vi "Begin.vi"(8 "error in":errorcluster) -> (0 "error out":errorcluster)   [LabVIEW 2020]
doc: "Called before other user functions, this VI is expected to open initial I/O refnums, load in file data, and do all program initialization. Notice that the <B>error out</B> terminal is simply used for data flow. Wiring it to other structures or subVIs ensures that this VI runs first."
uses:
  <vilib>/Rock Robotics/WPI/ThirdParty/Phoenix-LabVIEW/Pigeon2/controls/CTRE_Phoenix_Pigeon2_Configurables.ctl
  <vilib>/Rock Robotics/WPI/DriverStation/WPI_DriverStationRobotMode2.ctl
  <vilib>/Rock Robotics/WPI/Joystick/WPI_JoystickDeviceEnum.ctl
  <vilib>/Rock Robotics/WPI/SafetyOutput/WPI_SafetyOutputConfigMenu.ctl
  <vilib>/Rock Robotics/SystemInterfaces/DIO/FPGA_DIOChannel.ctl
  <vilib>/Rock Robotics/WPI/Solenoid/WPI_SolenoidChannel.ctl
  Robot Global Data.vi
  <vilib>/Rock Robotics/Network Tables/NT Write String Array.vi
  <vilib>/Rock Robotics/WPI/RobotDrive/WPI_RobotDriveOpen2MotorWithExistingMotors.vi
  <vilib>/Rock Robotics/WPI/Switch/WPI_SwitchOpenLimit.vi
  <vilib>/Rock Robotics/WPI/Solenoid/WPI_SolenoidOpenDouble.vi
panel:
  in  "Pigeon2 Configurables":T1
  in  "error in 2":errorcluster
  out "error out 2":errorcluster
  # "Yaw Angle needed to reach the current orientation in degrees"
  # "Configures the mounting pose of the Pigeon2\nThis is the yaw-pitch-roll teh Pigeon2 underwent to get to its current orientation,\n referenced from the robot's point of view\nThis is only necessary if the Pigeon2 is mounted at an exotic angle near the gimbal lock point or not forward.\nIf the pigeon is relatively flat and pointed forward, this is not needed"
  # "Pitch Angle needed to reach the current orientation in degrees"
  # "Roll Angle needed to reach the current orientation in degrees"
  # "Disables the temperature compensation\nfrom the Pigeon2. It is recommended that\nthis remains false"
  # "Disables the no-motion calibration from the\nPigeon2. It is recommended that this \nremains false"
  # "Enables the compass for Pigeon2\nThis is not recommended for any indoor robotics"
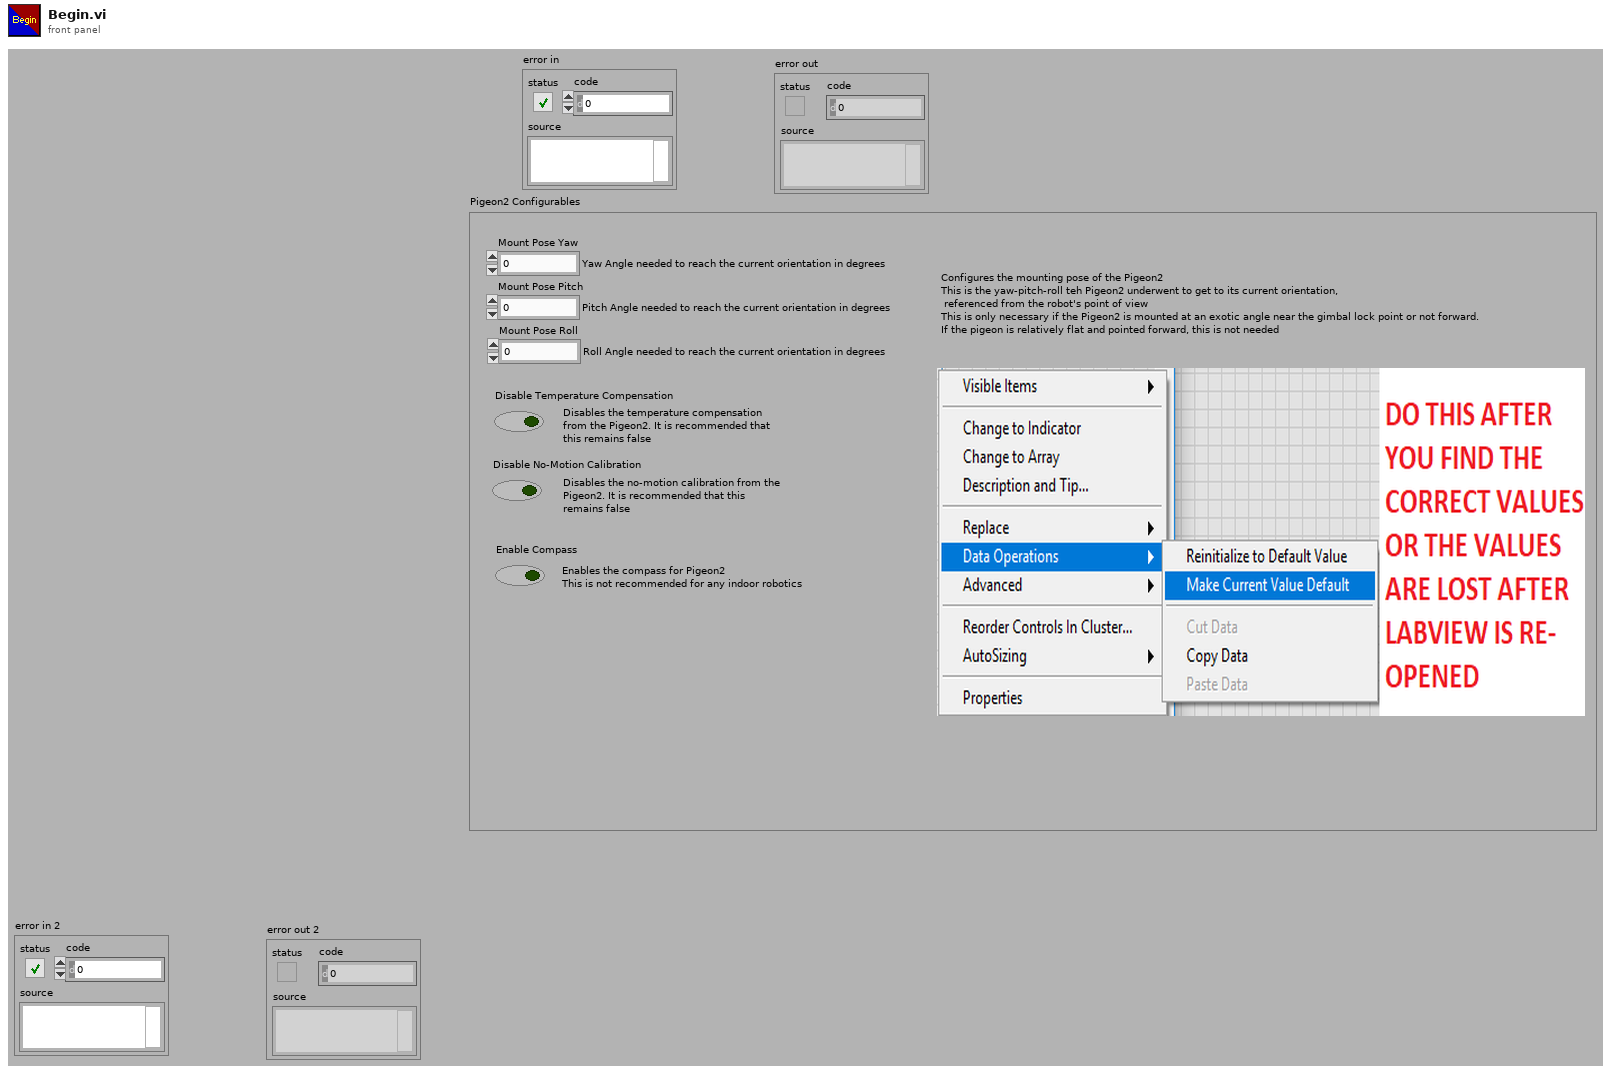
[diagram p1: front panel]
types:
  T1 = typedef "CTRE_Phoenix_Pigeon2_Configurables.ctl" = cluster{"Mount Pose Yaw":dbl, "Mount Pose Pitch":dbl, "Mount Pose Roll":dbl, "Disable Temperature Compensation":bool, "Disable No-Motion Calibration":bool, "Enable Compass":bool}
  T2 = typedef "WPI_SolenoidChannel.ctl" = enum8{"Solenoid 0", "Solenoid 1", "Solenoid 2", "Solenoid 3", "Solenoid 4", "Solenoid 5", "Solenoid 6", "Solenoid 7", "Solenoid 8", "Solenoid 9", "Solenoid 10", "Solenoid 11", "Solenoid 12", "Solenoid 13", "Solenoid 14", "Solenoid 15", "Invalid"}
  T3 = typedef "FPGA_DIOChannel.ctl" = enum8{"DIO 0", "DIO 1", "DIO 2", "DIO 3", "DIO 4", "DIO 5", "DIO 6", "DIO 7", "DIO 8", "DIO 9", "DIO MXP 0", "DIO MXP 1", "DIO MXP 2", "DIO MXP 3", "DIO MXP 4", "DIO MXP 5", "DIO MXP 6", "DIO MXP 7", "DIO MXP 8", "DIO MXP 9", "DIO MXP 10", "DIO MXP 11", "DIO MXP 12", "DIO MXP 13", "DIO MXP 14", "DIO MXP 15", "SPI Port CS1", "SPI Port CS2", "SPI Port CS3", "SPI Port MISO", "SPI Port MOSI", "Invalid"}
  T4 = typedef "WPI_JoystickDeviceEnum.ctl" = enum16{"USB 0", "USB 1", "USB 2", "USB 3", "USB 4", "USB 5"}
  T5 = typedef "WPI_SafetyOutputConfigMenu.ctl" = enum16{"Enable", "Disable"}
  T6 = typedef "WPI_DriverStationRobotMode2.ctl" = enum16{"Autonomous Disabled", "Autonomous Enabled", "Teleop Disabled", "Teleop Enabled", "Disconnected", "Finish", "Test Disabled", "Test Enabled", "Emergency Stopped"}
  T7 = typedef "WPI_JoystickDevRef.ctl" = cluster{"Device":T4}
  T8 = typedef "CTRE_PigeonIMU_DeviceRef.ctl" = cluster{"DeviceStatus":errorcluster, "Device Number":u8, "Type":T9, "Device ID":u32, "Handle":u64, "UsageFrame":u32, "Library Path":path}
  T9 = typedef "CTRE_PigeonIMU_ConnectionType.ctl" = u32
  T10 = typedef "WPI_SwitchDevRef.ctl" = cluster{"DevStatus":errorcluster, "DIO Channel":T3, "CntIndex":T11, "Normally Closed":bool}
  T11 = typedef "FPGA_CounterCtrSystemIndex.ctl" = enum8{"Ctr 0", "Ctr 1", "Ctr 2", "Ctr 3", "Ctr 4", "Ctr 5", "Ctr 6", "Ctr 7", "Invalid"}
  T12 = typedef "WPI_MotorControlDeviceRef.ctl" = cluster{"DeviceStatus":errorcluster, "Type":T13, "PWM":cluster{"PWM Channel":T14, "DeadBand":T15}, "CAN":cluster{"Device Number":u8, "SetOutput VI Ref":variant, "GetOutput VI Ref":variant, "Enable VI Ref":variant, "Disable VI Ref":variant, "Data":variant}, "Invert":bool, "DIO PWM":cluster{"PWM \"Enable\" Channel":T14, "DIOChannel":T3, "PWM Rate":dbl}}
  T13 = typedef "WPI_MotorControlType.ctl" = enum16{"PWM", "CAN", "DIO PWM"}
  T14 = typedef "FPGA_DIOPWMChannel.ctl" = enum8{"PWM 0", "PWM 1", "PWM 2", "PWM 3", "PWM 4", "PWM 5", "PWM 6", "PWM 7", "PWM 8", "PWM 9", "PWM MXP 0", "PWM MXP 1", "PWM MXP 2", "PWM MXP 3", "PWM MXP 4", "PWM MXP 5", "PWM MXP 6", "PWM MXP 7", "PWM MXP 8", "PWM MXP 9", "Invalid"}
  T15 = typedef "WPI_PWMDeadband.ctl" = cluster{"Name":string, "maxPositivePwm":i32, "minPositivePwm":i32, "centerPwm":i32, "maxNegativePwm":i32, "minNegativePwm":i32, "angularRange":u16}
  T16 = typedef "WPI_RobotDriveDevRef.ctl" = cluster{"DevStatus":errorcluster, "Motors[]":T12[], "Square Inputs":bool, "Max Output":dbl}
  T17 = typedef "WPI_SolenoidDevRef.ctl" = cluster{"DevStatus":errorcluster, "Pneumatics Control Module":u8, "Forward Solenoid Channel":T2, "Reverse Solenoid Channel":T2}
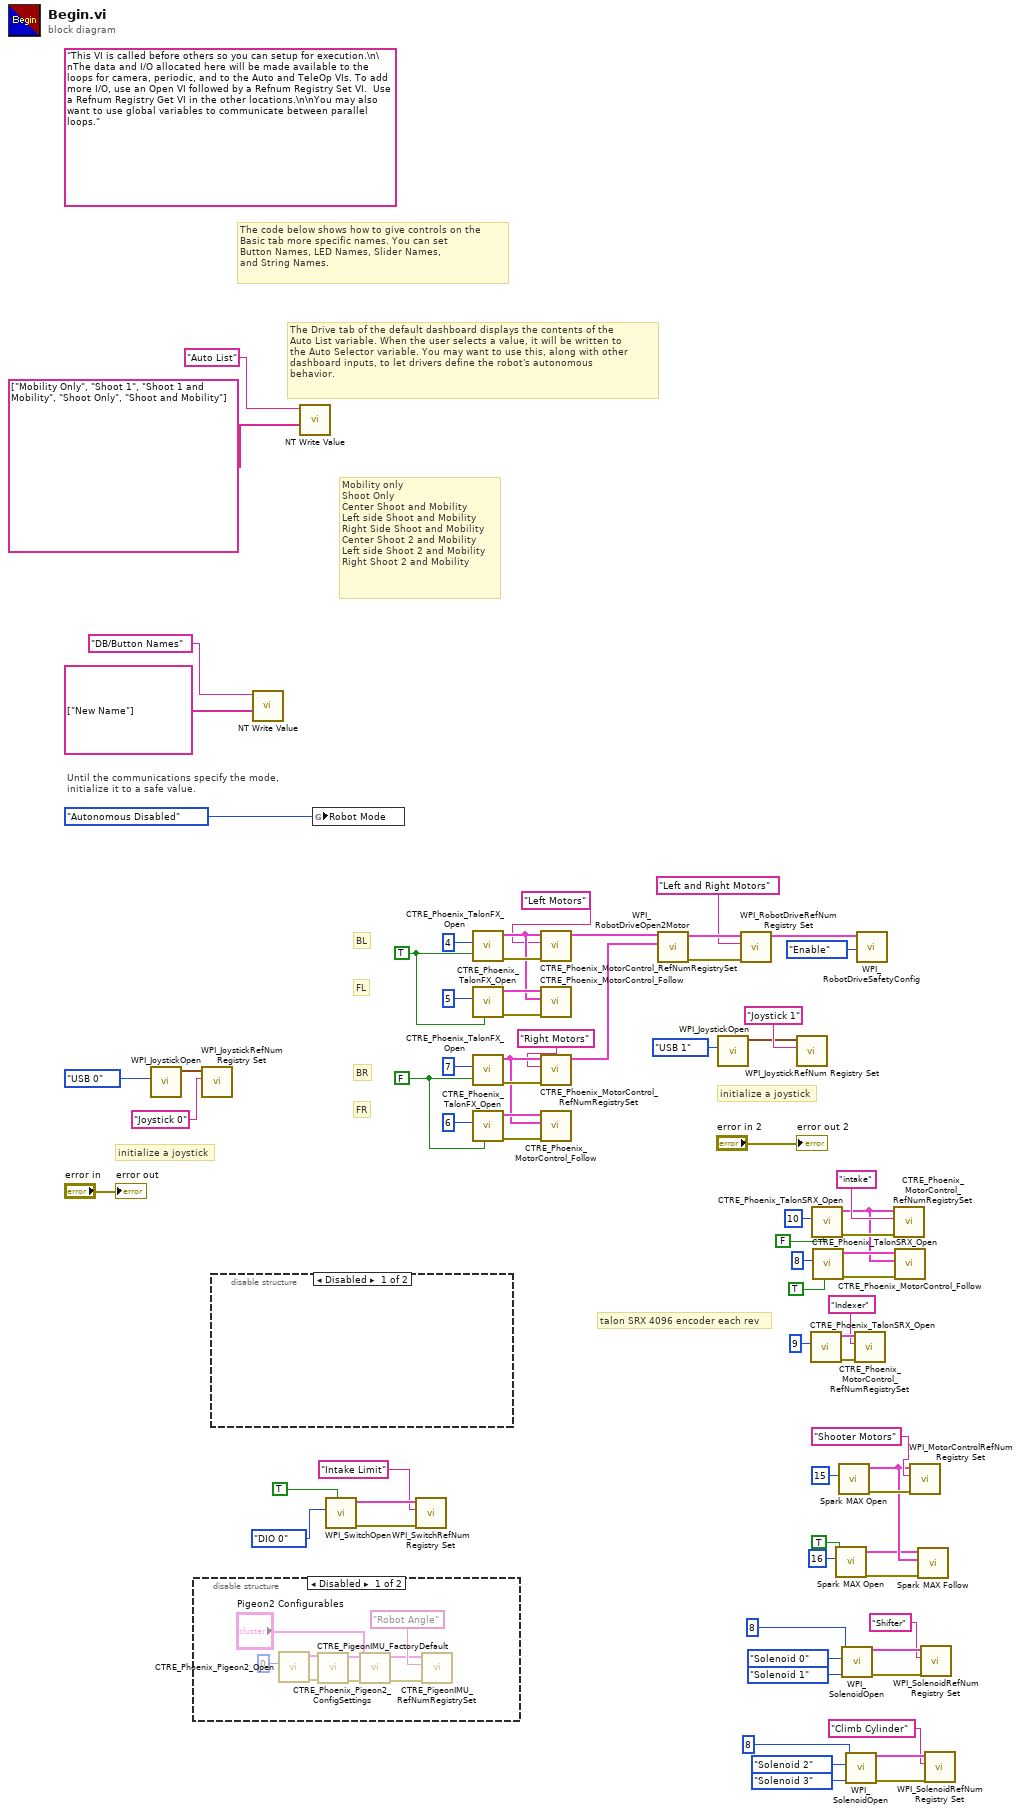
[diagram p0: block diagram]
diagram:
  w21 = TRUE ("Invert")
  w22 = FALSE ("Invert")
  (unwired) "This VI is called before others so you can setup for execution.\n\nThe data and I/O allocated here will be made available to the loops for camera, periodic, and to the Auto and TeleOp VIs. To add more I/O, use an Open VI followed by a Refnum Registry Set VI.  Use a Refnum Registry Get VI in the other locations.\n\nYou may also want to use global variables to communicate between parallel loops."
  # "Mobility only\nShoot Only\nCenter Shoot and Mobility\nLeft side Shoot and Mobility\nRight Side Shoot and Mobility\nCenter Shoot 2 and Mobility\nLeft side Shoot 2 and Mobility\nRight Shoot 2 and Mobility"
  # "talon SRX 4096 encoder each rev"
  # "FL"
  # "BL"
  # "BR"
  # "FR"
  # "initialize a joystick"
  # "The Drive tab of the default dashboard displays the contents of the\nAuto List variable. When the user selects a value, it will be written to\nthe Auto Selector variable. You may want to use this, along with other\ndashboard inputs, to let drivers define the robot's autonomous\nbehavior."
  # "The code below shows how to give controls on the\nBasic tab more specific names. You can set\nButton Names, LED Names, Slider Names,\nand String Names."
  # "initialize a joystick"
  # "Until the communications specify the mode,\ninitialize it to a safe value."
  n1 = call <vilib>:"WPI_JoystickOpen.vi"("JoystickDevice"=WPI_JoystickDeviceEnum."USB 0") -> ("JoystickDevRef"=w72:T7)  [unwired: 10 in]
  n2 = disable-structure shown="Disabled" {
    frame Disabled {
      n3 = call <vilib>:"CTRE_Phoenix_Pigeon2_Open.vi"("Device Number"=u8 0) -> ("error out"=w76:errorcluster, "PigeonIMUDevRef"=w77:T8)  [unwired: 9 in]
      n4 = call <vilib>:"CTRE_PigeonIMU_FactoryDefault.vi"("error in"=w76, "PigeonIMUDevRef"=w77) -> ("error out"=w78:errorcluster, "PigeonIMUDevRef"=w79:T8)  [unwired: 8 in]
      n5 = call <vilib>:"CTRE_Phoenix_Pigeon2_ConfigSettings.vi"("error in (no error)"=w78, "Pigeon2 Configurables"="Pigeon2 Configurables", "PigeonIMUDevRef 2"=w79) -> ("error out"=w81:errorcluster, "PigeonIMUDevRef"=w82:T8)  [unwired: 7 in]
      n6 = call <vilib>:"CTRE_PigeonIMU_RefNumRegistrySet.vi"("error in (no error)"=w81, "refnum name"="Robot Angle", "PigeonIMUDevRef"=w82) -> ()  [unwired: 7 in, 2 out]
    }
    frame Enabled {
    }
  }
  n7 = call <vilib>:"WPI_JoystickRefNum Registry Set.vi"("refnum name"="Joystick 0", "JoystickDevRef"=w72) -> ()  [unwired: 8 in, 2 out]
  n8 = disable-structure shown="Disabled" {
    frame Disabled {
    }
    frame Enabled {
    }
  }
  n9 = call-poly <vilib>:"NT Write Value.vi"("value"=string[] ["New Name"], "name"="DB/Button Names" ("Name")) -> ()  [unwired: 9 in, 1 out]
  n10 = call-poly <vilib>:"NT Write Value.vi"("value"=string[] ["Mobility Only", "Shoot 1", "Shoot 1 and Mobility", "Shoot Only", "Shoot and Mobility"] ("String Array"), "name"="Auto List" ("Name")) -> ()  [unwired: 9 in, 1 out]
  n11 = global write "Robot Global Data.vi" "Robot Mode"(WPI_DriverStationRobotMode2."Autonomous Disabled" ("Robot Mode")) -> ()
  n12 = call-poly <vilib>:"WPI_SwitchOpen.vi"("Normally Closed"=TRUE, "DIO Channel"=FPGA_DIOChannel."DIO 0") -> ("error out"=w16:errorcluster, "SwitchDevRef"=w17:T10)  [unwired: 8 in]
  n13 = call <vilib>:"WPI_SwitchRefNum Registry Set.vi"("error in (no error)"=w16, "refnum name"="Intake Limit", "SwitchDevRef"=w17) -> ()  [unwired: 7 in, 2 out]
  n14 = call <vilib>:"CTRE_Phoenix_TalonFX_Open.vi"("Invert"=w21, "Device Number"=u8 4) -> ("error out"=w36:errorcluster, "PhoenixMotorControlDevRef"=w34:T12)  [unwired: 8 in]
  n15 = call <vilib>:"CTRE_Phoenix_TalonFX_Open.vi"("Invert"=w21, "Device Number"=u8 5) -> ("error out"=w39:errorcluster, "PhoenixMotorControlDevRef"=w35:T12)  [unwired: 8 in]
  n16 = call <vilib>:"CTRE_Phoenix_TalonFX_Open.vi"("Invert"=w22, "Device Number"=u8 7) -> ("error out"=w30:errorcluster, "PhoenixMotorControlDevRef"=w28:T12)  [unwired: 8 in]
  n17 = call <vilib>:"CTRE_Phoenix_TalonFX_Open.vi"("Invert"=w22, "Device Number"=u8 6) -> ("error out"=w33:errorcluster, "PhoenixMotorControlDevRef"=w29:T12)  [unwired: 8 in]
  n18 = call <vilib>:"CTRE_Phoenix_MotorControl_RefNumRegistrySet.vi"("error in (no error)"=w36, "refnum name"="Left Motors", "PhoenixMotorControlDevRef"=w34) -> ("PhoenixMotorControlDevRef"=w27:T12)  [unwired: 7 in, 1 out]
  n19 = call <vilib>:"CTRE_Phoenix_MotorControl_Follow.vi"("error in (no error)"=w39, "Master Controller to Follow"=w34, "PhoenixMotorControlDevRef"=w35) -> ()  [unwired: 7 in, 2 out]
  n20 = call <vilib>:"CTRE_Phoenix_MotorControl_RefNumRegistrySet.vi"("error in (no error)"=w30, "refnum name"="Right Motors", "PhoenixMotorControlDevRef"=w28) -> ("PhoenixMotorControlDevRef"=w26:T12)  [unwired: 7 in, 1 out]
  n21 = call <vilib>:"CTRE_Phoenix_MotorControl_Follow.vi"("error in (no error)"=w33, "Master Controller to Follow"=w28, "PhoenixMotorControlDevRef"=w29) -> ()  [unwired: 7 in, 2 out]
  n22 = call-poly <vilib>:"WPI_RobotDriveOpen2Motor.vi"("Right Motor Dev Ref"=w26, "Left Motor Dev Ref"=w27) -> ("error out"=w46:errorcluster, "RobotDriveDevRef"=w47:T16)  [unwired: 3 in, 5 out]
  n23 = call <vilib>:"WPI_JoystickOpen.vi"("JoystickDevice"=WPI_JoystickDeviceEnum."USB 1") -> ("JoystickDevRef"=w42:T7)  [unwired: 10 in]
  n24 = call <vilib>:"WPI_RobotDriveRefNum Registry Set.vi"("error in (no error)"=w46, "refnum name"="Left and Right Motors", "RobotDriveDevRef"=w47) -> ("RobotDriveDevRef"=w45:T16)  [unwired: 1 in, 7 out]
  n25 = call <vilib>:"WPI_JoystickRefNum Registry Set.vi"("refnum name"="Joystick 1", "JoystickDevRef"=w42) -> ()  [unwired: 8 in, 2 out]
  n26 = call <vilib>:"CTRE_Phoenix_TalonSRX_Open.vi"("Device Number"=u8 9) -> ("error out"=w57:errorcluster, "PhoenixMotorControlDevRef"=w56:T12)  [unwired: 9 in]
  n27 = call <vilib>:"CTRE_Phoenix_TalonSRX_Open.vi"("Invert"=FALSE, "Device Number"=u8 10) -> ("error out"=w53:errorcluster, "PhoenixMotorControlDevRef"=w20:T12)  [unwired: 8 in]
  n28 = call <vilib>:"CTRE_Phoenix_TalonSRX_Open.vi"("Invert"=TRUE, "Device Number"=u8 8) -> ("error out"=w50:errorcluster, "PhoenixMotorControlDevRef"=w49:T12)  [unwired: 8 in]
  n29 = call <vilib>:"Spark MAX Open.vi"("Invert"=TRUE, "Device Number"=u8 16) -> ("error out"=w59:errorcluster, "MotorControlDeviceRef"=w60:T12)  [unwired: 8 in]
  n30 = call <vilib>:"Spark MAX Open.vi"("Device Number"=u8 15) -> ("error out"=w65:errorcluster, "MotorControlDeviceRef"=w61:T12)  [unwired: 9 in]
  n31 = call-poly <vilib>:"WPI_SolenoidOpen.vi"("Reverse Solenoid Channel"=WPI_SolenoidChannel."Solenoid 1", "Forward Solenoid Channel"=WPI_SolenoidChannel."Solenoid 0", "Pneumatics Device (def)"=u8 8) -> ("error out"=w9:errorcluster, "SolenoidDevRef"=w10:T17)  [unwired: 7 in]
  n32 = call-poly <vilib>:"WPI_SolenoidOpen.vi"("Reverse Solenoid Channel"=WPI_SolenoidChannel."Solenoid 3", "Forward Solenoid Channel"=WPI_SolenoidChannel."Solenoid 2", "Pneumatics Device (def)"=u8 8) -> ("error out"=w4:errorcluster, "SolenoidDevRef"=w5:T17)  [unwired: 7 in]
  n33 = call <vilib>:"CTRE_Phoenix_MotorControl_RefNumRegistrySet.vi"("error in (no error)"=w57, "refnum name"="Indexer", "PhoenixMotorControlDevRef"=w56) -> ()  [unwired: 7 in, 2 out]
  n34 = call <vilib>:"WPI_RobotDriveSafetyConfig.vi"("mode"=WPI_SafetyOutputConfigMenu."Enable", "RobotDriveDevRef"=w45) -> ()  [unwired: 8 in, 2 out]
  n35 = call <vilib>:"CTRE_Phoenix_MotorControl_RefNumRegistrySet.vi"("error in (no error)"=w53, "refnum name"="intake", "PhoenixMotorControlDevRef"=w20) -> ()  [unwired: 7 in, 2 out]
  n36 = call <vilib>:"CTRE_Phoenix_MotorControl_Follow.vi"("error in (no error)"=w50, "Master Controller to Follow"=w20, "PhoenixMotorControlDevRef"=w49) -> ()  [unwired: 7 in, 2 out]
  n37 = call <vilib>:"WPI_MotorControlRefNum Registry Set.vi"("error in (no error)"=w65, "refnum name"="Shooter Motors", "MotorControlDevRef"=w61) -> ()  [unwired: 7 in, 2 out]
  n38 = call <vilib>:"Spark MAX Follow.vi"("error in (no error)"=w59, "Master Controller"=w61, "MotorControlDeviceRef"=w60) -> ()  [unwired: 7 in, 2 out]
  n39 = call <vilib>:"WPI_SolenoidRefNum Registry Set.vi"("error in (no error)"=w9, "refnum name"="Shifter", "SolenoidDevRef"=w10) -> ()  [unwired: 7 in, 2 out]
  n40 = call <vilib>:"WPI_SolenoidRefNum Registry Set.vi"("error in (no error)"=w4, "refnum name"="Climb Cylinder", "SolenoidDevRef"=w5) -> ()  [unwired: 7 in, 2 out]
  "error out" <- "error in"
  "error out 2" <- "error in 2"
